vi "LVLM - Slave Sender.vi"   [LabVIEW 2010]
uses:
  <vilib>/NXT/Block Support/HWPage.SensorType.ctl
  <vilib>/NXT/Block Support/HWPage.SensorMode.ctl
  <vilib>/NXT/Block Support/NXT_InputPort.ctl
  <vilib>/NXT/Dual Mode Library/Sensors/i2c_sensors_big.vi
types:
  T1 = typedef "NXT_InputPort.ctl" = u8
  T2 = typedef "HWPage.SensorType.ctl" = u8
  T3 = typedef "HWPage.SensorMode.ctl" = u8
  T4 = typedef "LVHSConnector.ctl" = cluster{"Hardware":string, "Flattened String":string}
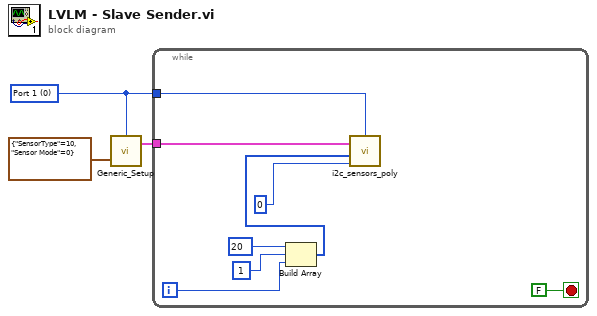
[diagram p0: block diagram]
diagram:
  w1 = T1 0 items=["Port 1", "Port 2", "Port 3", "Port 4"] ("Port")
  n1 = call <vilib>:"Generic_Setup.vi"("Sensor Setup"=cluster{"SensorType":T2, "Sensor Mode":T3} {"SensorType"=10, "Sensor Mode"=0}, "Port"=w1) -> ("NXT"=w2:T4)  [unwired: 1 in, 1 out]
  n2 = while {
    tunnel: w2 -> [w10]
    tunnel: w1 -> [w9]
    i -> [w5]
    stop <- FALSE stop-if-true
    n3 = Build Array(u8 20, 1, w5) -> (w4:i32[])
    n4 = call-poly <vilib>:"i2c_sensors_poly.vi"("Return Length"=u8 0, "Bytes to Write"=w4, "NXT"=w10, "Port"=w9) -> ()  [unwired: 1 in, 3 out]
  }
